vi "Drum Pad Mixer Example.vi"() -> ()   [LabVIEW 2020]
uses:
  Mixer/Mixer/Mixer.lvclass
  Mixer/Mixer/Polymorphic VIs/Channel Load (Path).vi
panel:
  in  "Stop":bool
  in  "Sample Pack":u16(ring) items=["Dataflow_G", "Misc", "Trap 1"]
  in  "Play 16":bool caption="V"
  in  "Play 15":bool caption="C"
  in  "Play 14":bool caption="X"
  in  "Play 13":bool caption="Z"
  in  "Play 12":bool caption="F"
  in  "Play 11":bool caption="D"
  in  "Play 10":bool caption="S"
  in  "Play 9":bool caption="A"
  in  "Play 8":bool caption="R"
  in  "Play 7":bool caption="E"
  in  "Play 6":bool caption="W"
  in  "Play 5":bool caption="Q"
  in  "Play 4":bool caption="4"
  in  "Play 3":bool caption="3"
  in  "Play 2":bool caption="2"
  in  "Play 1":bool caption="1"
  # "Instructions:\n1. Run the VI.\n2. Select an audio file to play using the path control.\n3. Use the controls to change the visualizer color and size.\n4. Press the Stop button to stop playback."
  # "G"
  # "-Audio"
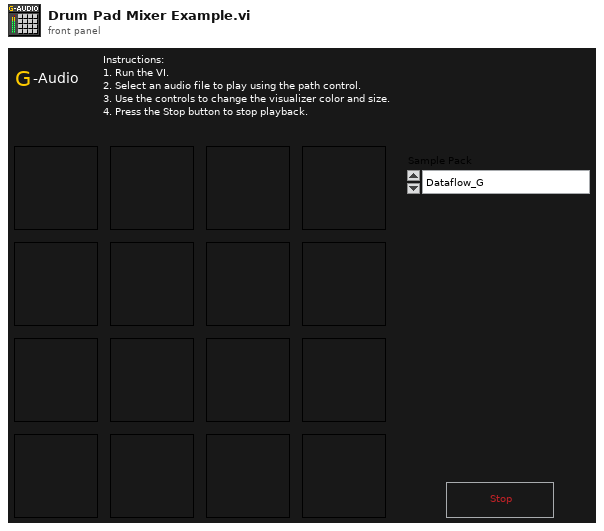
[diagram p1: front panel]
types:
  T1 = typedef "G-Audio.lvlib/Channel.lvclass/Channel Status.ctl" = cluster{"Frame":u64, "State":T2, "Volume":dbl}
  T2 = typedef "G-Audio.lvlib/Channel.lvclass/Channel State.ctl" = enum16{"Empty", "Error", "Loading", "Loaded", "Stopped", "Paused", "Playing", "Retrigger"}
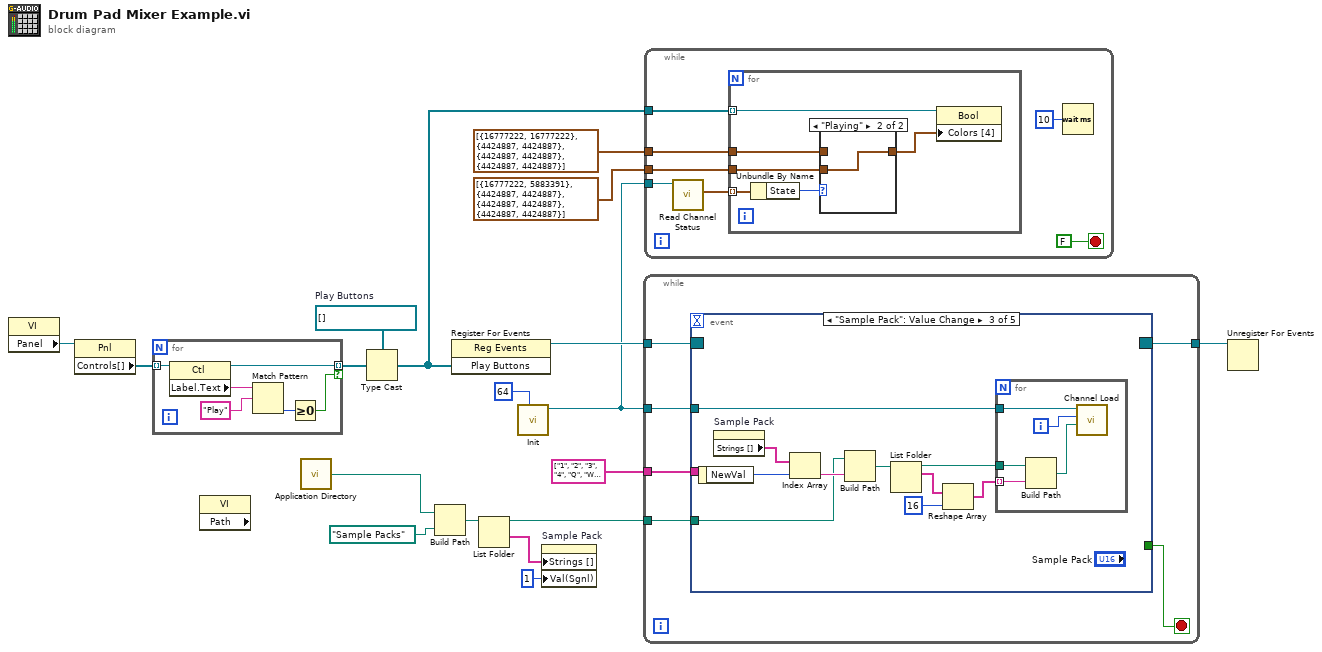
[diagram p0: block diagram]
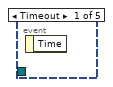
[diagram p3: hidden frame]
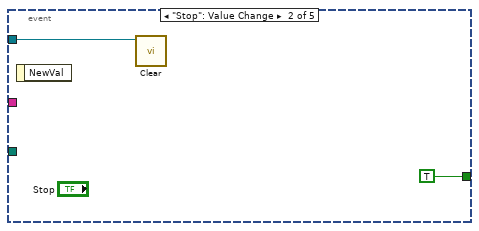
[diagram p4: hidden frame]
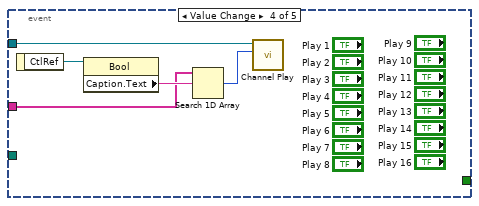
[diagram p5: hidden frame]
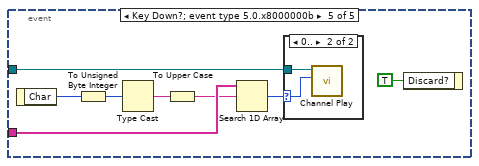
[diagram p6: hidden frame]
diagram:
  w18 = refnum<vi>[] []  # Play Buttons
  n1 = property class="VI"() -> ("Panel"=w10:refnum<vi>)  [unwired: 2 in, 2 out]
  n2 = property class="Pnl"(reference=w10) -> ("Controls[]"=w9:refnum<vi>[])  [unwired: 1 in, 2 out]
  n3 = for {
    tunnel: w9 -> [w24] mode=indexing
    tunnel: [w23] -> w7 mode=indexing if=w19
    n4 = property class="Ctl"(reference=w24) -> (reference out=w23:refnum<vi>, "Label.Text"=w22:string)  [unwired: 1 in, 1 out]
    n5 = Match Pattern(string=w22, regular expression="Play") -> (offset past match=w20:i32)  [unwired: 1 in, 3 out]
    n6 = Greater Or Equal To 0?(x=w20) -> (x >= 0?=w19:bool)
  }
  n7 = property class="VI" props=["Path"]() -> ()  [unwired: 2 in, 3 out]
  n8 = call <vilib>:"Application Directory.vi"() -> ("Application Directory"=w1:path)
  n9 = Type Cast(type=w18, x=w7) -> (*(type *) &x=w6:refnum<vi>[])
  n10 = Build Path(base path=w1, name or relative path=path "Sample Packs") -> (appended path=w14:path)
  n11 = register-events(w6) -> (reference out=w17:refnum<event-registration>)  [unwired: 2 in, 1 out]
  n12 = List Folder(path=w14) -> (path out=w12:path, folder names=w13:string[])  [unwired: 3 in, 2 out]
  n13 = call "Init.vi"("Playback Size (4096)"=64) -> ("Mixer out"=w2:refnum<class "Mixer.lvclass">)  [unwired: 9 in, 1 out]
  n14 = property on="Sample Pack" class="Ring (strict)"("Strings []"=w13, "Val(Sgnl)"=u16 1 ("Value (Signaling)")) -> ()  [unwired: 2 in, 2 out]
  n15 = while {
    tunnel: w17 -> [w30]
    tunnel: w2 -> [w29]
    tunnel: string[] ["1", "2", "3", "4", "Q", "W", "E", "R", "A", "S", "D", "F", "Z", "X", "C", "V"] -> [w28]
    tunnel: w12 -> [w27]
    tunnel: [w25] -> w8
    stop <- w26 stop-if-true
    n16 = event shown="[2] \"Sample Pack\": Value Change" {
      selector: w30 -> [_ _ _ _ _]
      dyn-events: [_ _ _ _ _] -> w25
      timeout: _ -> [_ _ _ _ _]
      tunnel: w29 -> [_ w32 w34 w51 w60]
      tunnel: w28 -> [_ _ _ w49 w58]
      tunnel: w27 -> [_ _ w40 _ _]
      tunnel: [_ TRUE _ _ _] -> w26
      event Timeout {
        n17 = event-data() -> ()  [unwired: 1 in, 1 out]
      }
      event "Stop": Value Change {
        n18 = event-data() -> ()  [unwired: 1 in, 1 out]
        n19 = call "Clear.vi"("Mixer in"=w32) -> ()  [unwired: 10 in, 1 out]
      }
      event "Sample Pack": Value Change {
        n20 = event-data() -> ("NewVal"=w42:u16)  [unwired: 1 in]
        n21 = property on="Sample Pack" class="Ring (strict)"() -> ("Strings []"=w39:string[])  [unwired: 2 in, 2 out]
        n22 = Index Array(array=w39, index=w42) -> (element=w41:string)
        n23 = Build Path(base path=w40, name or relative path=w41) -> (appended path=w38:path)
        n24 = List Folder(path=w38) -> (path out=w35:path, filenames=w37:string[])  [unwired: 3 in, 2 out]
        n25 = Reshape Array(w37, 16 ("dimension size")) -> (w36:string[])
        n26 = for {
          tunnel: w36 -> [w47] mode=indexing
          tunnel: w35 -> [w46]
          tunnel: w34 -> [w45]
          i -> [w44]
          n27 = Build Path(base path=w46, name or relative path=w47) -> (appended path=w43:path)
          n28 = call-poly "Channel Load.vi"("Path"=w43, "Channel Index"=w44, "Mixer in"=w45) -> ()  [unwired: 7 in, 2 out]
        }
      }
      event Value Change {
        n29 = event-data() -> ("CtlRef"=w52:refnum<vi>)  [unwired: 1 in]
        n30 = property class="Bool"(reference=w52) -> ("Caption.Text"=w50:string)  [unwired: 1 in, 2 out]
        n31 = Search 1D Array(1D array=w49, element=w50) -> (index of element=w48:i32)  [unwired: 1 in]
        n32 = call "Channel Play.vi"("Channel Index"=w48, "Mixer in"=w51) -> ()  [unwired: 8 in, 2 out]
      }
      event Key Down?; event type 5.0.x8000000b {
        n33 = event-data() -> ("Char"=w59:i16)  [unwired: 1 in]
        n34 = To Unsigned Byte Integer(number=w59) -> (unsigned 8bit integer=w55:u8)
        n35 = Type Cast(x=w55) -> (*(type *) &x=w53:string)  [unwired: 1 in]
        n36 = To Upper Case(1:w53) -> (0:w56:string)
        n37 = Search 1D Array(1D array=w58, element=w56) -> (index of element=w54:i32)  [unwired: 1 in]
        n38 = case shown="0.." w54 {
          selector: w54 -> [_ w61]
          tunnel: w60 -> [_ w62]
          frame Default {
          }
          frame 0.. {
            n39 = call "Channel Play.vi"("Channel Index"=w61, "Mixer in"=w62) -> ()  [unwired: 8 in, 2 out]
          }
        }
        n40 = event-data("Discard?"=TRUE) -> ()  [unwired: 1 in, 1 out]
      }
    }
  }
  n41 = while {
    tunnel: w2 -> [w69]
    tunnel: w6 -> [w67]
    tunnel: cluster{u32, u32}[] [{16777222, 16777222}, {4424887, 4424887}, {4424887, 4424887}, {4424887, 4424887}] ("Colors [4]") -> [w66]
    tunnel: cluster{u32, u32}[] [{16777222, 5883391}, {4424887, 4424887}, {4424887, 4424887}, {4424887, 4424887}] ("Colors [4]") -> [w65]
    stop <- FALSE stop-if-true
    n42 = call "Read Channel Status.vi"("Mixer in"=w69) -> ("Channel Status"=w68:T1[])  [unwired: 8 in, 2 out]
    n43 = for {
      tunnel: w68 -> [w75] mode=indexing
      tunnel: w67 -> [w73] mode=indexing
      tunnel: w66 -> [w72]
      tunnel: w65 -> [w70]
      n44 = Unbundle By Name(w75) -> ("State"=w74:T2)
      n45 = case shown="\"Playing\"" w74 {
        tunnel: w72 -> [w76 _]
        tunnel: [w76 w77] -> w71
        tunnel: w70 -> [_ w77]
        frame Default {
        }
        frame "Playing" {
        }
      }
      n46 = property class="Bool"(reference=w73, "Colors [4]"=w71) -> ()  [unwired: 1 in, 2 out]
    }
    n47 = Wait (ms)(milliseconds to wait=u32 10) -> ()  [unwired: 1 out]
  }
  n48 = Unregister For Events(event registration refnum=w8) -> ()  [unwired: 1 in, 1 out]
